vi "Handle Error.vi"(7 "Stop on Unhandled Error (T)":bool=TRUE, 8 "error in":errorcluster, 11 "Logger.PGSQL":refnum<class "Logger.PGSQL.lvclass">) -> (0 "handling error":errorcluster, 2 "Unhandled error":errorcluster, 3 "Logger.PGSQL out":refnum<class "Logger.PGSQL.lvclass">)   [LabVIEW 2019, in "Logger.PGSQL.lvlib" / "Logger.PGSQL.lvclass"]
doc: "JKI State Machine Objects (SMO) 1.0.0.11\nJKI - JKI\nCopyright (c) 2016, JKI"
uses:
  Logger.PGSQL.lvclass
  Logger.PGSQL.lvclass/Logger.PGSQL.ctl
  <userlib>/LevyLab/Logger/Logger/Logger.lvclass
  <userlib>/LevyLab/LV-Data/LV-Data.PG/LV-Data.PGSQL.lvclass
panel:
  # "For instructions on how to use the JKI State Machine Objects, examples and video tutorials, visit:\nhttp://jki.net/state-machine-objects/\n\nJKI State Machine Objects™\nhttp://jki.net/state-machine-objects/\nCopyright (C) 2005-2015, JKI <info@jki.net>\nALL RIGHTS RESERVED"
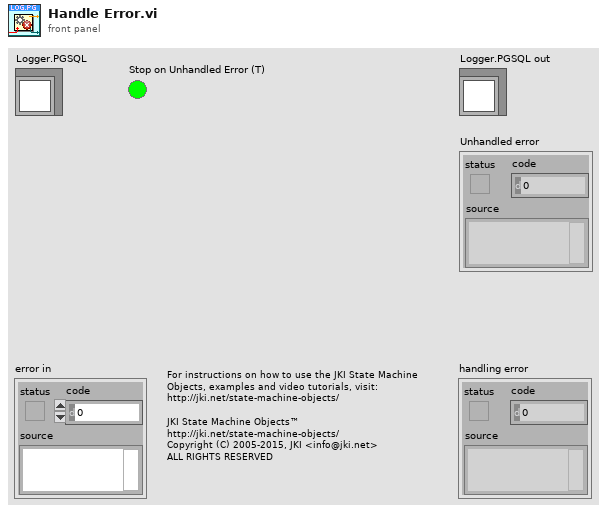
[diagram p1: front panel]
types:
  T1 = enum16{"unconfigured", "disconnected", "connected"}
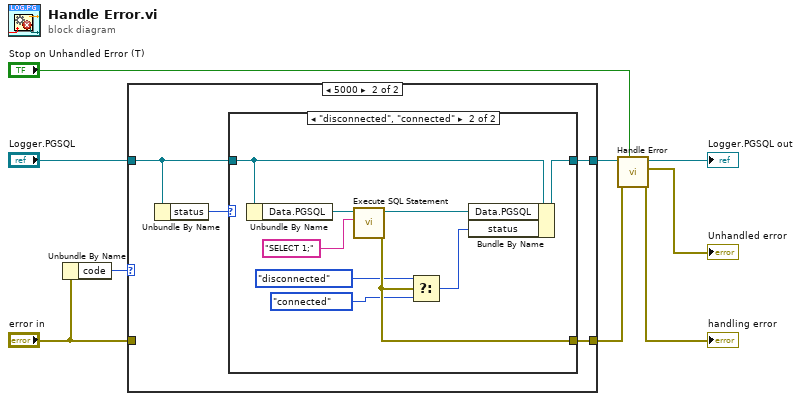
[diagram p0: block diagram]
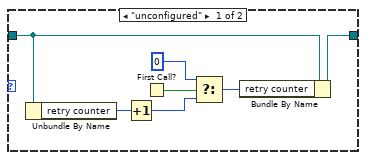
[diagram p3: hidden frame]
diagram:
  n1 = Unbundle By Name("error in") -> ("code"=w4:i32)
  n2 = case shown="5000" w4 {
    tunnel: [w11 w12] -> w7
    tunnel: "error in" -> [w11 _]
    tunnel: "Logger.PGSQL" -> [w10 w14]
    tunnel: [w10 w15] -> w1
    frame Default {
    }
    frame 5000 {
      n3 = Unbundle By Name(w14) -> ("status"=w13:T1)
      n4 = case shown="\"disconnected\", \"connected\"" w13 {
        tunnel: w14 -> [w19 w28]
        tunnel: [w17 w29] -> w15
        tunnel: [_ w26] -> w12
        frame "unconfigured" {
          n5 = Unbundle By Name(w19) -> ("retry counter"=w21:i32)
          n6 = Increment(x=w21) -> (x+1=w20:i32)
          n7 = First Call?() -> (First Call?: T/F=w22:bool)
          n8 = Select(t=0, s=w22, f=w20) -> (s? t:f=w18:i32)
          n9 = Bundle By Name(cluster=w19, "retry counter"=w18) -> (w17:refnum<class "Logger.PGSQL.lvclass">)
        }
        frame "disconnected", "connected" {
          n10 = Unbundle By Name(w28) -> ("Data.PGSQL"=w31:refnum<class "LV-Data.PGSQL.lvclass">)
          n11 = call <userlib>:"Execute SQL Statement.vi"("SQL string"="SELECT 1;", "Data.PGQL in"=w31) -> ("error out"=w26:errorcluster, "Data.PGSQL out"=w30:refnum<class "LV-Data.PGSQL.lvclass">)  [unwired: 7 in, 1 out]
          n12 = Select(t=T1."disconnected" ("status"), s=w26, f=T1."connected" ("status")) -> (s? t:f=w23:T1)
          n13 = Bundle By Name(cluster=w28, "Data.PGSQL"=w30, "status"=w23) -> (w29:refnum<class "Logger.PGSQL.lvclass">)
        }
      }
    }
  }
  n14 = call-parent "Handle Error.vi"("Stop on Unhandled Error (T)"="Stop on Unhandled Error (T)", "error in"=w7, "SMO"=w1) -> ("handling error"=→"handling error":errorcluster, "Unhandled error"=→"Unhandled error":errorcluster, "SMO out"=→"Logger.PGSQL out":refnum<class "Logger.PGSQL.lvclass">)  [unwired: 6 in]
